vi "Plotter_Transmit_Parameter.vi"(8 "error in (no error)":errorcluster, 11 "Globals":T1) -> ()   [LabVIEW 2017]
uses:
  Controls/Plotter_Globals.ctl
  Classes/ADCP.lvclass
  Controls/Plotter_Queues.ctl
  Controls/Plotter_Queue_Command_and_Data.ctl
  Controls/Plotter_Commands.ctl
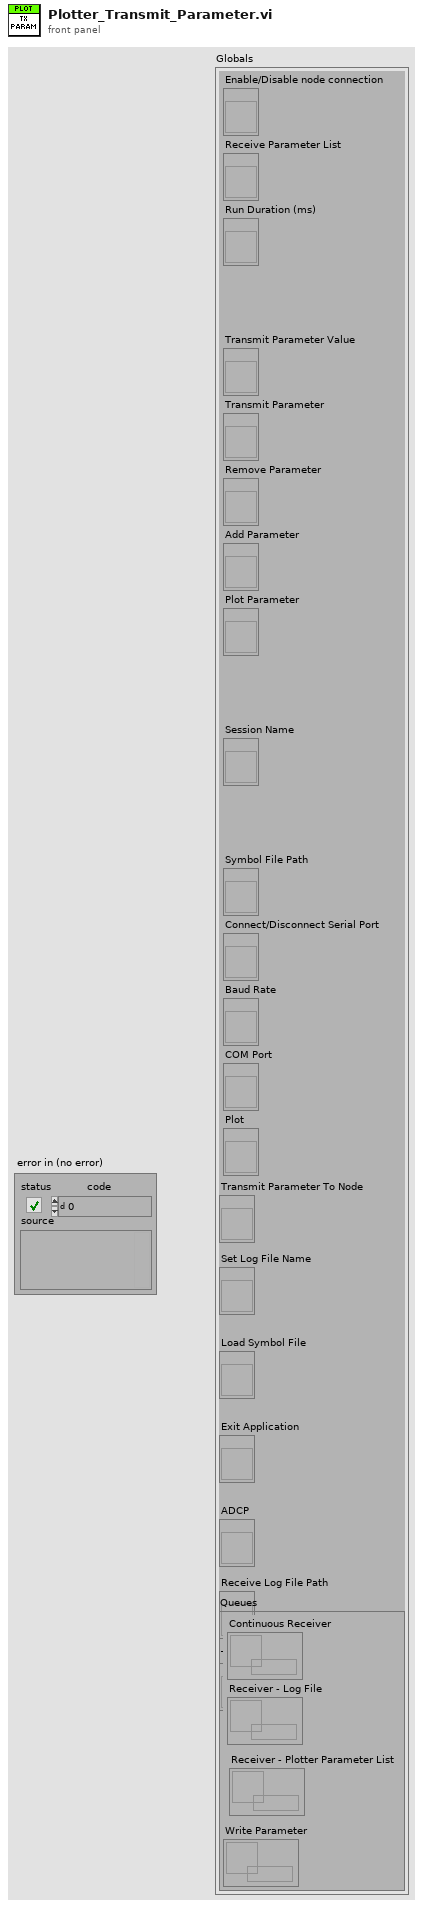
[diagram p1: front panel]
types:
  T1 = typedef "Plotter_Globals.ctl" = cluster{"Enable/Disable node connection":refnum<vi>, "Receive Parameter List":refnum<vi>, "Run Duration (ms)":refnum<vi>, "Transmit Parameter Value":refnum<vi>, "Transmit Parameter":refnum<vi>, "Remove Parameter":refnum<vi>, "Add Parameter":refnum<vi>, "Plot Parameter":refnum<vi>, "Session Name":refnum<vi>, "Symbol File Path":refnum<vi>, "Connect/Disconnect Serial Port":refnum<vi>, "Baud Rate":refnum<vi>, "COM Port":refnum<vi>, "Plot":refnum<vi>, "Transmit Parameter To Node":refnum<vi>, "Set Log File Name":refnum<vi>, "Load Symbol File":refnum<vi>, "Exit Application":refnum<vi>, "ADCP":refnum<vi>, "Transmit Log File Path":refnum<vi>, "Receive Log File Path":refnum<vi>, "Queues":T2}
  T2 = typedef "Plotter_Queues.ctl" = cluster{"Continuous Receiver":refnum<queue>, "Receiver - Log File":refnum<queue>, "Receiver - Plotter Parameter List":refnum<queue>, "Write Parameter":refnum<queue>}
  T3 = typedef "Plotter_Queue_Command_and_Data.ctl" = cluster{"Commands":T4, "Data":variant}
  T4 = typedef "Plotter_Commands.ctl" = enum16{"Idle", "Cont_RX_Open_Node", "Cont_RX_Flush_Serial_Port", "Cont_Rx_Log_Write", "Plot_Update", "Exit"}
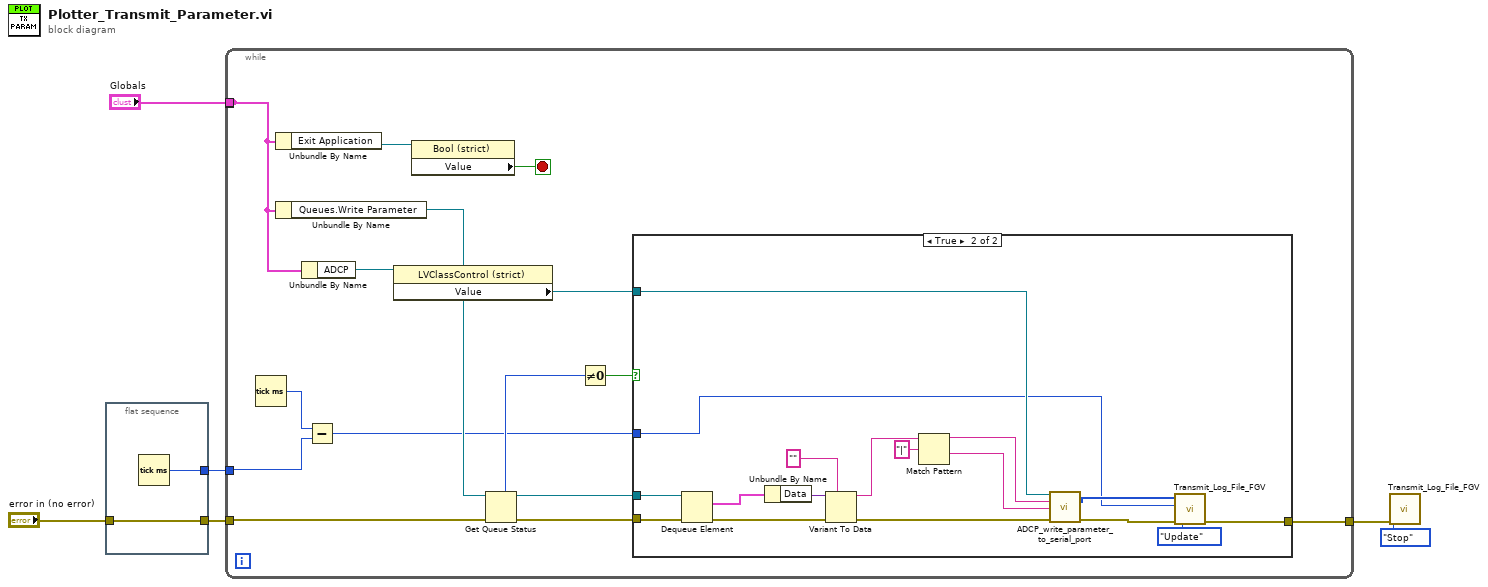
[diagram p0: block diagram]
diagram:
  n1 = flat-sequence {
    tunnel: "error in (no error)" -> [w8]
    tunnel: [w8] -> w4
    tunnel: [w7] -> w3
    frame #0 {
      n2 = Tick Count (ms)() -> (millisecond timer value=w7:u32)
    }
  }
  n3 = while {
    tunnel: [w14] -> _
    tunnel: "Globals" -> [w14]
    tunnel: w4 -> [w23]
    tunnel: [w17] -> w2
    tunnel: w3 -> [w10]
    stop <- w15 stop-if-true
    n4 = Tick Count (ms)() -> (millisecond timer value=w11:u32)
    n5 = Unbundle By Name(w14) -> ("Exit Application"=w16:refnum<vi>)
    n6 = Unbundle By Name(w14) -> ("Queues.Write Parameter"=w22:refnum<queue>)
    n7 = Unbundle By Name(w14) -> ("ADCP"=w13:refnum<vi>)
    n8 = Subtract(x=w11, y=w10) -> (x-y=w9:u32)
    n9 = property class="LVClassControl (strict)"(reference=w13) -> ("Value"=w12:refnum<class "ADCP.lvclass">)  [unwired: 1 in, 2 out]
    n10 = property class="Bool (strict)"(reference=w16) -> ("Value"=w15:bool)  [unwired: 1 in, 2 out]
    n11 = Get Queue Status(queue=w22, error in (no error)=w23) -> (queue out=w18:refnum<queue>, error out=w20:errorcluster, # elements in queue=w21:i32)  [unwired: 1 in, 5 out]
    n12 = Not Equal To 0?(x=w21) -> (x != 0?=w19:bool)
    n13 = case shown="True" w19 {
      tunnel: w20 -> [w24 w41]
      tunnel: w18 -> [_ w40]
      tunnel: [w24 w28] -> w17
      tunnel: w12 -> [_ w38]
      tunnel: w9 -> [_ w25]
      frame False {
      }
      frame True {
        n14 = Dequeue Element(queue=w40, error in (no error)=w41) -> (element=w39:T3, error out=w37:errorcluster)  [unwired: 1 in, 2 out]
        n15 = Unbundle By Name(w39) -> ("Data"=w35:variant)
        n16 = Variant To Data(error in=w37, type="", Variant=w35) -> (data=w33:string, error out=w36:errorcluster)
        n17 = Match Pattern(string=w33, regular expression="|") -> (before substring=w31:string, after substring=w30:string)  [unwired: 1 in, 2 out]
        n18 = call "ADCP_write_parameter_to_serial_port.vi"("ADCP In"=w38, "Parameter name"=w31, "Parameter value"=w30, "error in (no error)"=w36) -> ("Processed bytes"=w26:u8[], "error out"=w29:errorcluster)  [unwired: 8 in, 2 out]
        n19 = call "Transmit_Log_File_FGV.vi"("error in (no error)"=w29, "Command"=enum16{"Initialize", "Update", "Stop"}."Update", "Time (ms)"=w25, "Processed bytes"=w26) -> ("error out"=w28:errorcluster)  [unwired: 6 in, 1 out]
      }
    }
  }
  n20 = call "Transmit_Log_File_FGV.vi"("error in (no error)"=w2, "Command"=enum16{"Initialize", "Update", "Stop"}."Stop") -> ()  [unwired: 8 in, 2 out]
